vi "set_MC_box_overlay.vi"(6 "RAPS array in":T2(array[cluster]), 8 "error in (no error)":errorcluster, 10 "Reference Image in":T1(plugin-control) caption="2011_04_13__16_49_46h__channel01", 11 "TrajectoryMH100122AODRAPS in":refnum<class "TrajectoryMH100122AODRAPS.lvclass">) -> (0 "error out":errorcluster, 2 "Reference Image out":T1, 3 "TrajectoryMH100122AODRAPS out":refnum<class "TrajectoryMH100122AODRAPS.lvclass">, 4 "number of MC points out":i32)   [LabVIEW 2010, in "TrajectoryMH100122AODRAPS.lvclass"]
uses:
  TrajectoryMH100122AODRAPS.lvclass
  <vilib>/vision/Image Controls.llb/IMAQ Image.ctl
  TrajectoryMH100122AODRAPS.lvclass/TrajectoryMH100122AODRAPS.ctl
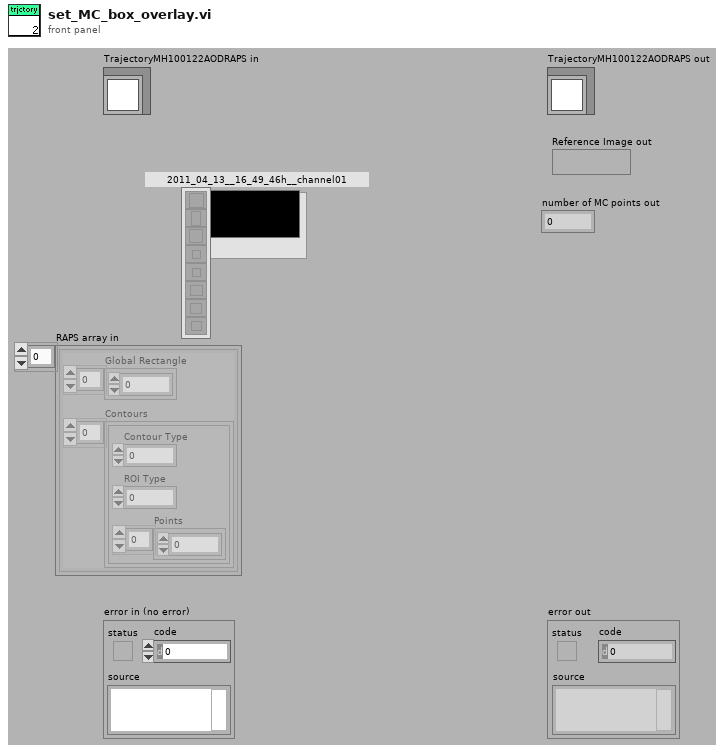
[diagram p1: front panel]
types:
  T1 = typedef "IMAQ Image.ctl" = refnum<image>
  T2 = cluster{"Global Rectangle":i32[], "Contours":cluster{"Contour Type":u32, "ROI Type":u32, "Points":i32[]}[]}[]
  T3 = cluster{"Contour Type":u32, "ROI Type":u32, "Points":i32[]}[]
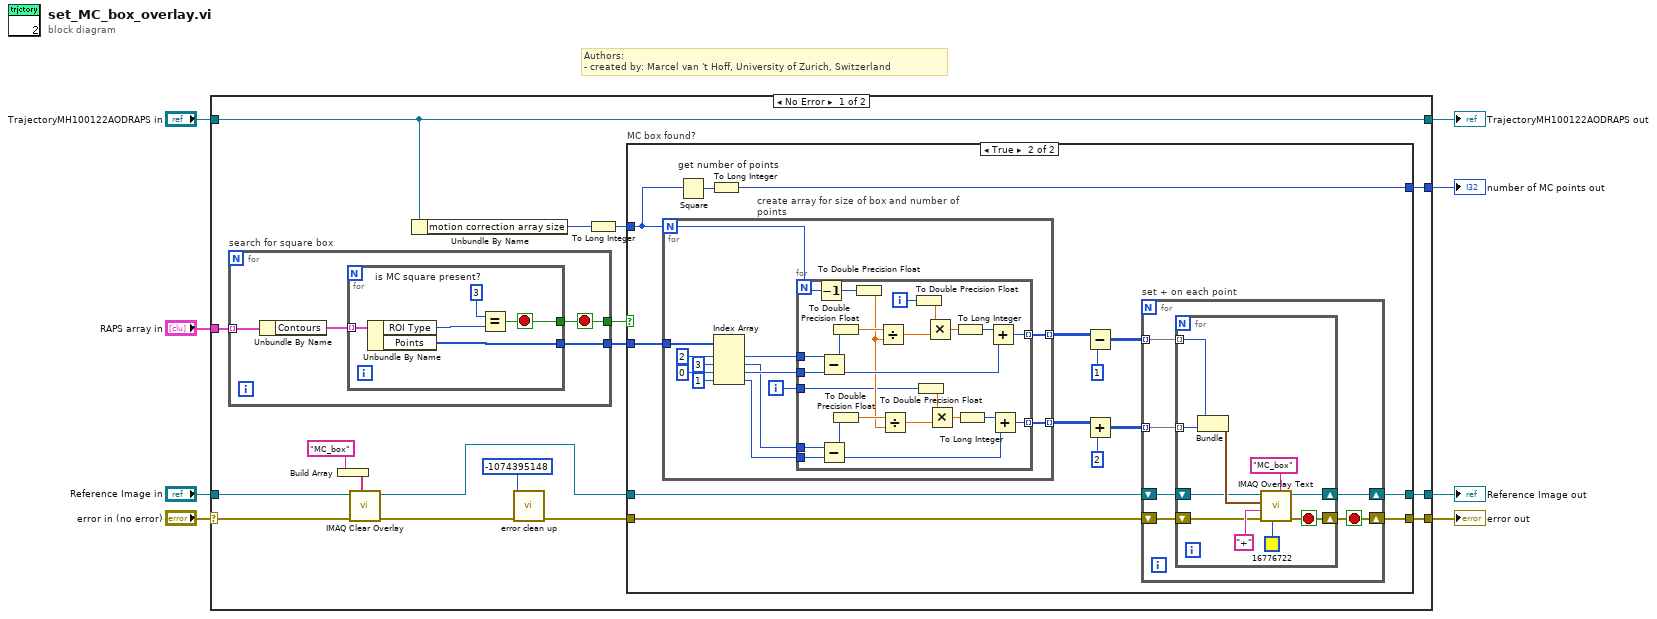
[diagram p0: block diagram]
diagram:
  # "Authors: \n- created by: Marcel van 't Hoff, University of Zurich, Switzerland"
  n1 = case shown="No Error" "error in (no error)" {
    selector: "error in (no error)" -> [w16 w105]
    tunnel: [w22 w105] -> w7
    tunnel: [w10 w104] -> w5
    tunnel: "TrajectoryMH100122AODRAPS in" -> [w10 w104]
    tunnel: "RAPS array in" -> [w25 _]
    tunnel: "Reference Image in" -> [w17 w103]
    tunnel: [w11 w103] -> w2
    tunnel: [w9 _] -> w1
    frame No Error {
      n2 = for "search for square box" {
        tunnel: w25 -> [w97] mode=indexing
        tunnel: [w95] -> w24
        tunnel: [w94] -> w23
        stop <- w95 stop-if-true
        n3 = Unbundle By Name(w97) -> ("Contours"=w96:T3)
        n4 = for {
          tunnel: w96 -> [w102] mode=indexing
          tunnel: [w99] -> w95
          tunnel: [w98] -> w94
          stop <- w99 stop-if-true
          w101 = u32 3  # is MC square present?
          n5 = Unbundle By Name(w102) -> ("ROI Type"=w100:u32, "Points"=w98:i32[])
          n6 = Equal?(x=w101, y=w100) -> (x = y?=w99:bool)
        }
      }
      n7 = Build Array("MC_box" ("Group")) -> (w18:string[])
      n8 = call "IMAQ Clear Overlay"("Groups"=w18, "error in (no error)"=w16, "Image"=w17) -> ("error out"=w15:errorcluster, "Image Out"=w13:T1)  [unwired: 7 in]
      n9 = Unbundle By Name(w10) -> ("motion correction array size"=w21:u8)
      n10 = call "error clean up.vi"("error in"=w15, "code in"=-1074395148 ("code")) -> ("error out"=w14:errorcluster)  [unwired: 9 in]
      n11 = To Long Integer(number=w21) -> (32bit integer=w20:i32)
      n12 = case "MC box found?" shown="True" w24 {
        tunnel: w23 -> [_ w41]
        tunnel: w14 -> [w27 w34]
        tunnel: [w27 w33] -> w22
        tunnel: w20 -> [_ w29]
        tunnel: w13 -> [w26 w32]
        tunnel: [w26 w31] -> w11
        tunnel: [_ w28] -> w9
        frame False {
        }
        frame True {
          n13 = for "create array for size of box and number of points" {
            N: w29 -> [w64]
            tunnel: w41 -> [w70]
            tunnel: [w69] -> w39 mode=indexing
            tunnel: [w61] -> w37 mode=indexing
            i -> [w58]
            n14 = Index Array(array=w70, index #1=2 ("index"), index #2=3 ("index"), index #3=0 ("index"), index #4=1 ("index")) -> (element #1=w66:i32, element #2=w60:i32, element #3=w65:i32, element #4=w59:i32)
            n15 = for {
              N: w64 -> [w92]
              tunnel: w66 -> [w85]
              tunnel: w65 -> [w84]
              tunnel: [w87] -> w69 mode=indexing
              tunnel: [w71] -> w61 mode=indexing
              tunnel: w60 -> [w75]
              tunnel: w59 -> [w74]
              tunnel: w58 -> [w72]
              i -> [w88]
              n16 = Decrement(x=w92) -> (x-1=w86:i32)
              n17 = Subtract(x=w85, y=w84) -> (x-y=w93:i32)
              n18 = Subtract(x=w75, y=w74) -> (x-y=w81:i32)
              n19 = To Double Precision Float(number=w93) -> (double precision float=w90:dbl)
              n20 = To Double Precision Float(number=w81) -> (double precision float=w79:dbl)
              n21 = To Double Precision Float(number=w86) -> (double precision float=w73:dbl)
              n22 = Divide(x=w90, y=w73) -> (x/y=w83:dbl)
              n23 = Divide(x=w79, y=w73) -> (x/y=w77:dbl)
              n24 = To Double Precision Float(number=w88) -> (double precision float=w82:dbl)
              n25 = To Double Precision Float(number=w72) -> (double precision float=w76:dbl)
              n26 = Multiply(x=w82, y=w83) -> (x*y=w91:dbl)
              n27 = Multiply(x=w76, y=w77) -> (x*y=w80:dbl)
              n28 = To Long Integer(number=w91) -> (32bit integer=w89:i32)
              n29 = To Long Integer(number=w80) -> (32bit integer=w78:i32)
              n30 = Add(x=w89, y=w84) -> (x+y=w87:i32)
              n31 = Add(x=w78, y=w74) -> (x+y=w71:i32)
            }
          }
          n32 = Square "get number of points"(x=w29) -> (x^2=w30:i32)
          n33 = To Long Integer(number=w30) -> (32bit integer=w28:i32)
          n34 = Subtract(x=w39, y=1 ("index")) -> (x-y=w40:i32[][])
          n35 = Add(x=w37, y=2 ("index 2")) -> (x+y=w38:i32[][])
          n36 = for "set + on each point" {
            tunnel: w40 -> [w47] mode=indexing
            tunnel: w38 -> [w46] mode=indexing
            shift-right: [w44] -> w33
            shift-left: w34 -> [w45]
            shift-right: [w42] -> w31
            shift-left: w32 -> [w43]
            stop <- w44 stop-if-true
            n37 = for {
              tunnel: w47 -> [w52] mode=indexing
              tunnel: w46 -> [w51] mode=indexing
              shift-right: [w53] -> w44
              shift-left: w45 -> [w54]
              shift-right: [w48] -> w42
              shift-left: w43 -> [w49]
              stop <- w53 stop-if-true
              n38 = Bundle(w52, w51) -> (w50:cluster{i32, i32})  [unwired: 1 in]
              n39 = call "IMAQ Overlay Text"("Group"="MC_box", "Text Color (black)"=u32 16776722, "error in (no error)"=w54, "String"="+", "Origin"=w50, "Image"=w49) -> ("error out"=w53:errorcluster, "Image Out"=w48:T1)  [unwired: 4 in]
            }
          }
        }
      }
    }
    frame Error {
    }
  }
  "error out" <- w7
  "TrajectoryMH100122AODRAPS out" <- w5
  "Reference Image out" <- w2
  "number of MC points out" <- w1
